vi "Find Changed Value.vi"(9 "Old Value":T1, 10 "New Value":T1, 11 "CtlRef":refnum<vi>) -> (2 "Value":bool, 3 "Target":string)   [LabVIEW 2019, in "DIG_IO.lvlib" / "DIG_IO.lvclass"]
uses:
  Library/DIG_IO.lvclass
  Custom Controls/Single_Bank.ctl
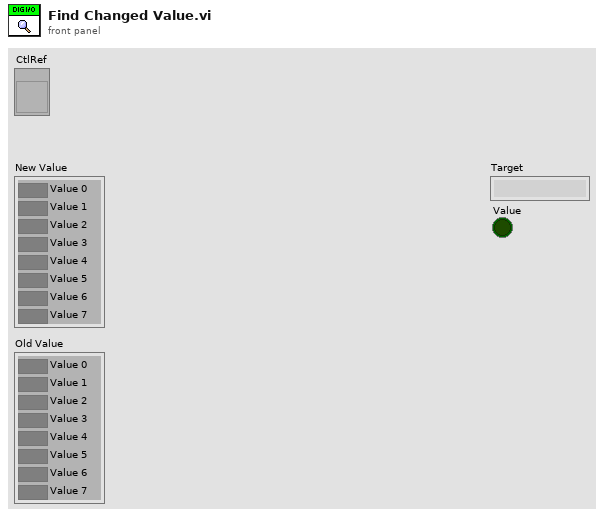
[diagram p1: front panel]
types:
  T1 = typedef "DIG_IO.lvlib/DIG_IO.lvclass/Single_Bank.ctl" = cluster{"Value 0":bool, "Value 1":bool, "Value 2":bool, "Value 3":bool, "Value 4":bool, "Value 5":bool, "Value 6":bool, "Value 7":bool}
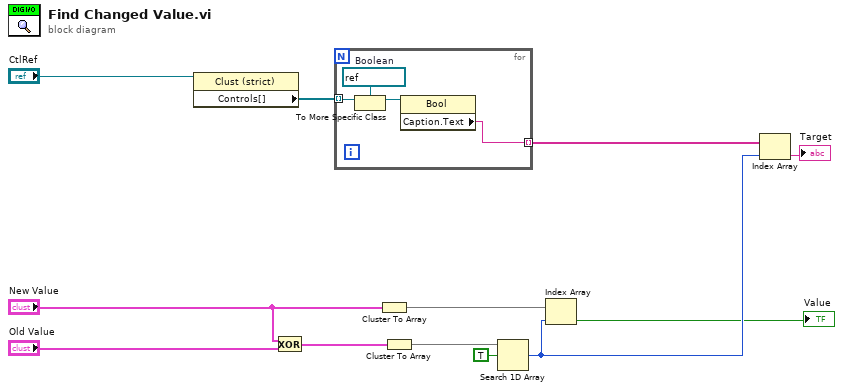
[diagram p0: block diagram]
diagram:
  n1 = property class="Clust (strict)"(reference="CtlRef") -> ("Controls[]"=w8:refnum<vi>[])  [unwired: 1 in, 2 out]
  n2 = Exclusive Or(1:"Old Value", 2:"New Value") -> (0:w12:T1)
  n3 = for {
    tunnel: w8 -> [w16] mode=indexing
    tunnel: [w13] -> w7 mode=indexing
    w14 = refnum<vi> refnum  # Boolean
    n4 = To More Specific Class(target class=w14, reference=w16) -> (specific class reference=w15:refnum<vi>)  [unwired: 1 in, 1 out]
    n5 = property class="Bool"(reference=w15) -> ("Caption.Text"=w13:string)  [unwired: 1 in, 2 out]
  }
  n6 = Cluster To Array(cluster="New Value") -> (array=w6:bool[])
  n7 = Cluster To Array(cluster=w12) -> (array=w11:bool[])
  n8 = Search 1D Array(1D array=w11, element=TRUE) -> (index of element=w5:i32)  [unwired: 1 in]
  n9 = Index Array(array=w6, index=w5) -> (element=→"Value":bool)
  n10 = Index Array(array=w7, index=w5) -> (element=→"Target":string)
